vi "fromStringSpectrum.vi"(1 "value":string[](array[string]), 2 "attribute name":string, 3 "device name":string) -> (0 "attribute value":T1={"device name"="", "attribute name"="", "quality value"=enum."VALID", "quality string"="", "timestamp"=0.0, "dim. x"=0, "dim. y"=0, "value"=[], "error code"=0, "error stack"=[], "data type"=enum."UNKNOWN_DATA_TYPE"})   [LabVIEW 2014, in "tango.lvlib"]
uses:
  tango.lvlib
  Common VIs/Typedefs/_AttributeValue_t.ctl
  Common VIs/Typedefs/_AttributeQuality_t.ctl
  Common VIs/Typedefs/_AttributeDataType_t.ctl
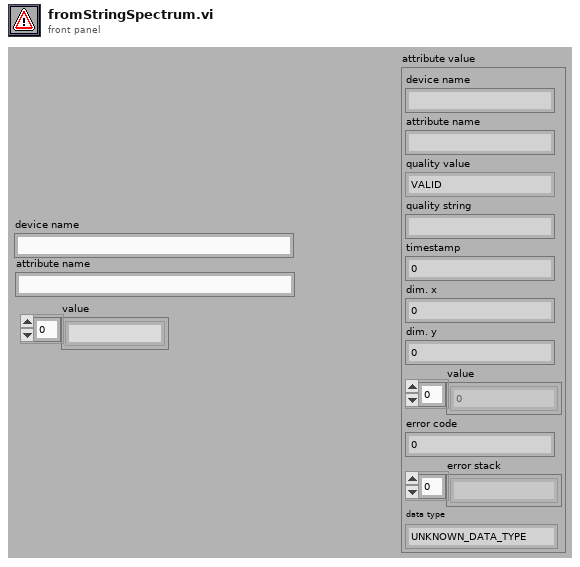
[diagram p1: front panel]
types:
  T1 = typedef "tango.lvlib/_AttributeValue_t.ctl" = cluster{"device name":string, "attribute name":string, "quality value":T2, "quality string":string, "timestamp":dbl, "dim. x":i32, "dim. y":i32, "value":u8[], "error code":i32, "error stack":string[], "data type":T3}
  T2 = typedef "tango.lvlib/_AttributeQuality_t.ctl" = enum16{"VALID", "INVALID", "ALARM", "CHANGING", "UNKNOWN_QUALITY"}
  T3 = typedef "tango.lvlib/_AttributeDataType_t.ctl" = enum16{"STATE_SCA", "STATE_SPE", "STATE_IMG", "STRING_SCA", "STRING_SPE", "STRING_IMG", "BOOL_SCA", "BOOL_SPE", "BOOL_IMG", "UCHAR_SCA", "UCHAR_SPE", "UCHAR_IMG", "SHORT_SCA", "SHORT_SPE", "SHORT_IMG", "USHORT_SCA", "USHORT_SPE", "USHORT_IMG", "LONG_SCA", "LONG_SPE", "LONG_IMG", "ULONG_SCA", "ULONG_SPE", "ULONG_IMG", "LONG64_SCA", "LONG64_SPE", "LONG64_IMG", "ULONG64_SCA", "ULONG64_SPE", "ULONG64_IMG", "FLOAT_SCA", "FLOAT_SPE", "FLOAT_IMG", "DOUBLE_SCA", "DOUBLE_SPE", "DOUBLE_IMG", "UNKNOWN_DATA_TYPE"}
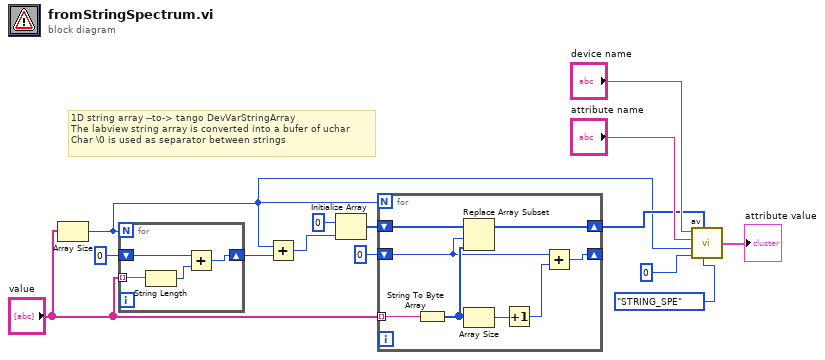
[diagram p0: block diagram]
diagram:
  # "1D string array --to-> tango DevVarStringArray\nThe labview string array is converted into a bufer of uchar\nChar \\0 is used as separator between strings"
  n1 = Array Size(array="value") -> (size(s)=w2:i32)
  n2 = for {
    N: w2 -> [_]
    tunnel: "value" -> [w17] mode=indexing
    shift-right: [w15] -> w6
    shift-left: 0 -> [w16]
    n3 = String Length(string=w17) -> (length=w18:i32)
    n4 = Add(x=w16, y=w18) -> (x+y=w15:i32)
  }
  n5 = Add(x=w2, y=w6) -> (x+y=w5:i32)
  n6 = Initialize Array(u8 0, w5) -> (w8:u8[])
  n7 = for {
    N: w2 -> [_]
    shift-right: [w23] -> w3
    shift-left: w8 -> [w25]
    tunnel: "value" -> [w26] mode=indexing
    shift-right: [w21] -> _
    shift-left: 0 -> [w19]
    n8 = String To Byte Array(string=w26) -> (unsigned byte array=w24:u8[])
    n9 = Replace Array Subset(array=w25, new element=w24, index=w19) -> (w23:u8[])
    n10 = Array Size(array=w24) -> (size(s)=w22:i32)
    n11 = Increment(x=w22) -> (x+1=w20:i32)
    n12 = Add(x=w19, y=w20) -> (x+y=w21:i32)
  }
  n13 = call "av.vi"("tango data type"=_AttributeDataType_t."STRING_SPE" ("Control"), "data"=w3, "dim. y"=0, "dim. x"=w2, "attribute name"="attribute name", "device name"="device name") -> ("attribute value"=→"attribute value":T1)
